vi "FTW-XML-Query-Elements.vi"(0 "XML Node":refnum<k20>, 5 "XPath Query":string, 11 "error in":errorcluster) -> (4 "XML Node out":refnum<k20>, 6 "Matching Nodes":refnum<k20>[](array[refnum]), 8 "Num Matches":i32, 15 "error out":errorcluster)   [LabVIEW 2013, in "XML.lvlib"]
uses:
  XML.lvlib
  DOMUserDefRef.dll
panel:
  # "Inputs"
  # "Outputs"
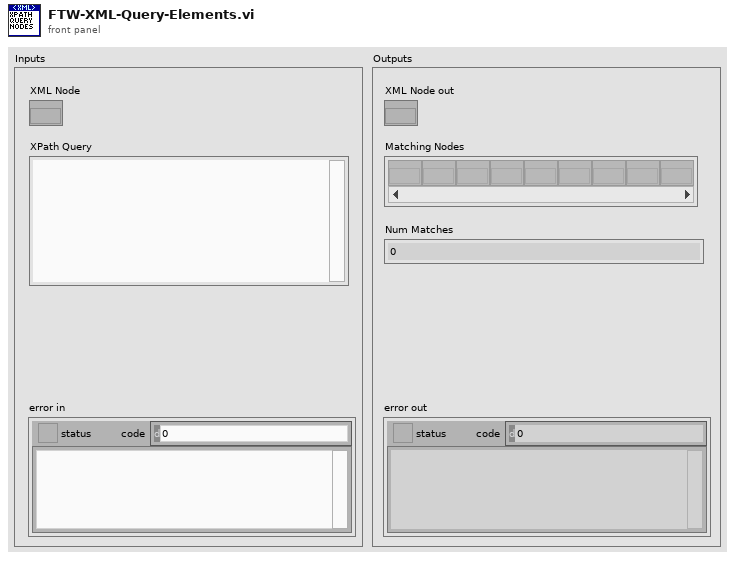
[diagram p1: front panel]
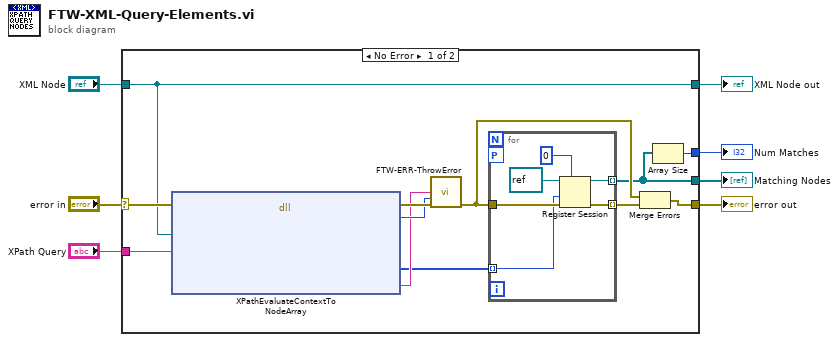
[diagram p0: block diagram]
diagram:
  n1 = case shown="No Error" "error in" {
    selector: "error in" -> [w19 w27]
    tunnel: [w10 w27] -> w7
    tunnel: "XML Node" -> [w16 w26]
    tunnel: [w16 w26] -> w4
    tunnel: "XPath Query" -> [w17 _]
    tunnel: [w9 _] -> w2
    tunnel: [w8 _] -> w1
    frame No Error {
      n2 = dll-call lib="DOMUserDefRef.*" fn="XPathEvaluateContextToNodeArray"(error in=w19, "Base Node"=w16, "XPath Query"=w17) -> (error out=w18:errorcluster, "Return"=w15:i32, "Matching Nodes"=w13:u64[], "Error String"=w14:string)  [unwired: 3 in, 4 out]
      n3 = call "FTW-ERR-ThrowError.vi"("Error Message"=w14, "Error Code"=w15, "error in"=w18) -> ("error out"=w12:errorcluster)  [unwired: 12 in]
      n4 = for {
        tunnel: w12 -> [w23]
        tunnel: [w22] -> w9 mode=indexing
        tunnel: w13 -> [w21] mode=indexing
        workers-P: _ -> [_]
        tunnel: [w20] -> w11 mode=indexing
        n5 = Register Session(7:0 ("cleanup mode (default to class = 0)"), 8:w23, 9:w21, 11:refnum<k20> refnum ("refnum")) -> (0:w20:errorcluster, 3:w22:refnum<k20>)  [unwired: 1 in]
      }
      n6 = Merge Errors(w12, w11) -> (w10:errorcluster)
      n7 = Array Size(array=w9) -> (size(s)=w8:i32)
    }
    frame Error {
    }
  }
  "error out" <- w7
  "XML Node out" <- w4
  "Matching Nodes" <- w2
  "Num Matches" <- w1
